vi "Open Sheet.vi"(8 "error in (no error)":errorcluster, 10 "Name (Sheet1)":string="Sheet1", 11 "Excel in":refnum<class "Excel.lvclass">) -> (0 "error out":errorcluster, 3 "Excel out":refnum<class "Excel.lvclass">)   [LabVIEW 2016, in "Excel.lvclass"]
doc: "Activates and shows a worksheet within the workbook referenced by the Excel input object.\n\nThis VI can be used to specify a particular worksheet to interact with and also to create new worksheets.\n\nIf a worksheet name is provided that sheet will be activated and shown within the workbook. If the worksheet does not exist within the workbook it will be created. If no sheet name is specified a default \"Sheet1\" is used and will also be created if not found in the workbook."
uses:
  Excel.lvclass
  Excel.lvclass/Excel.ctl
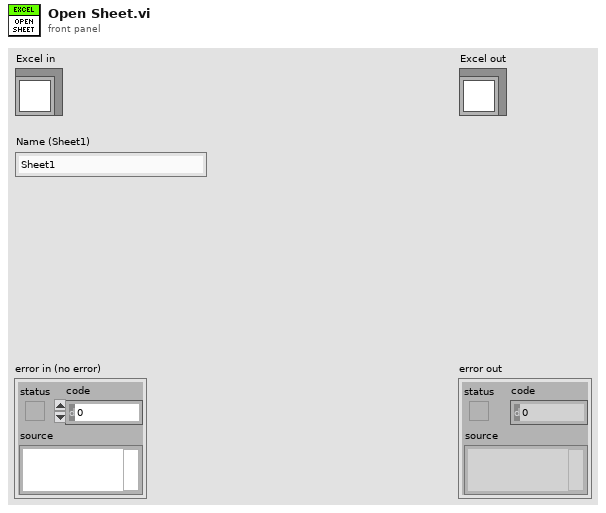
[diagram p1: front panel]
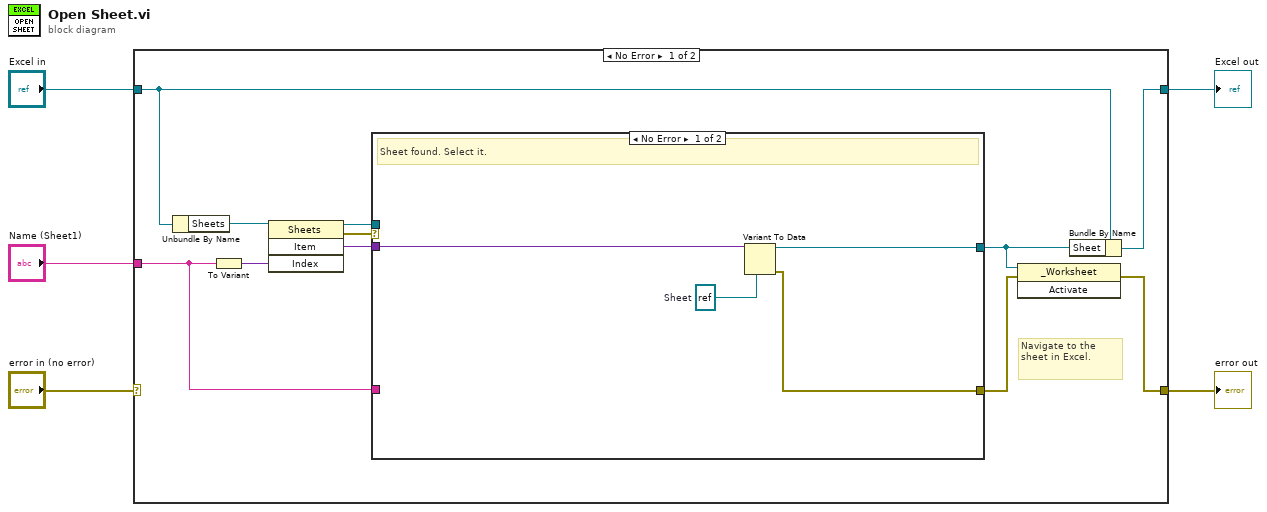
[diagram p0: block diagram]
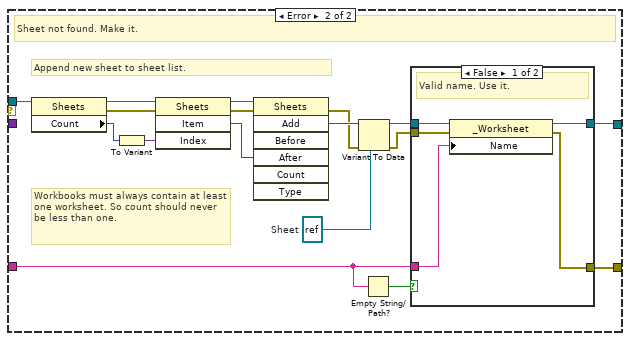
[diagram p2: hidden frame]
diagram:
  n1 = case shown="No Error" "error in (no error)" {
    selector: "error in (no error)" -> [_ w46]
    tunnel: [w6 w46] -> w4
    tunnel: [w9 w45] -> w2
    tunnel: "Excel in" -> [w10 w45]
    tunnel: "Name (Sheet1)" -> [w11 _]
    frame No Error {
      # "Navigate to the sheet in Excel."
      n2 = Unbundle By Name(w10) -> ("Sheets"=w16:refnum<k7>)
      n3 = To Variant(anything=w11) -> (Variant=w15:variant)
      n4 = invoke class="Sheets" method="Item"(reference=w16, "Index"=w15) -> (reference out=w12:refnum<k7>, error out=w13:errorcluster, "Item"=w14:variant)  [unwired: 2 in, 1 out]
      n5 = case shown="No Error" w13 {
        tunnel: w14 -> [w20 _]
        tunnel: w12 -> [_ w28]
        tunnel: [w18 w32] -> w8
        tunnel: w11 -> [_ w30]
        tunnel: [w17 w31] -> w7
        frame No Error {
          w19 = refnum<k7> refnum  # Sheet
          # "Sheet found. Select it."
          n6 = Variant To Data(type=w19, Variant=w20) -> (data=w18:refnum<k7>, error out=w17:errorcluster)  [unwired: 1 in]
        }
        frame Error {
          w35 = refnum<k7> refnum  # Sheet
          # "Workbooks must always contain at least one worksheet. So count should never be less than one."
          # "Append new sheet to sheet list."
          # "Sheet not found. Make it."
          n7 = property class="Sheets"(reference=w28) -> (reference out=w27:refnum<k7>, error out=w26:errorcluster, "Count"=w21:i32)  [unwired: 1 in]
          n8 = To Variant(anything=w21) -> (Variant=w22:variant)
          n9 = invoke class="Sheets" method="Item"(reference=w27, error in=w26, "Index"=w22) -> (reference out=w25:refnum<k7>, error out=w24:errorcluster, "Item"=w23:variant)  [unwired: 1 in, 1 out]
          n10 = invoke class="Sheets" method="Add"(reference=w25, error in=w24, "After"=w23) -> (error out=w36:errorcluster, "Add"=w37:variant)  [unwired: 4 in, 5 out]
          n11 = Variant To Data(error in=w36, type=w35, Variant=w37) -> (data=w34:refnum<k7>, error out=w33:errorcluster)
          n12 = Empty String/Path?(string/path=w30) -> (empty?=w29:bool)
          n13 = case shown="False" w29 {
            tunnel: w34 -> [w42 w44]
            tunnel: w33 -> [w41 w43]
            tunnel: w30 -> [w40 _]
            tunnel: [w39 w44] -> w32
            tunnel: [w38 w43] -> w31
            frame False {
              # "Valid name. Use it."
              n14 = property class="_Worksheet"(reference=w42, error in=w41, "Name"=w40) -> (reference out=w39:refnum<k7>, error out=w38:errorcluster)
            }
            frame True {
              # "Invalid name. Leave default."
            }
          }
        }
      }
      n15 = invoke class="_Worksheet" method="Activate"(reference=w8, error in=w7) -> (error out=w6:errorcluster)  [unwired: 1 in, 2 out]
      n16 = Bundle By Name(cluster=w10, "Sheet"=w8) -> (w9:refnum<class "Excel.lvclass">)
    }
    frame Error {
    }
  }
  "error out" <- w4
  "Excel out" <- w2
